vi "Keithley 6514 Resistance Config.vi"(0 "Resource In":refnum<visa-resource-name>, 1 "Check For SCPI Errors? (T)":bool=TRUE, 5 "range (autorange:0)":u16(ring) items=["autorange", "set min range", "set max range", "set man range value"], 7 "NPLC value (1.00)":dbl=1.0 min=0.01 max=10.0 step=0.01 format="%.2f", 9 "man range value (ohms) (210e3)":sgl=210000.0 min=0 max=2.1e+11 step=1 format="%^.2e", 11 "error in (no error)":T1, 12 "Autorange Upper Limit (ohms) (210e9)":sgl=210000000000.0 min=0 max=2.1e+11 step=1 format="%^.2e", 13 "Autorange Lower Limit (ohms) (2.1e3)":sgl=2100.0 min=0 max=2.1e+11 step=1 format="%^.2e", 14 "Driven Guard":bool) -> (4 "Resource Out (dupl)":refnum<visa-resource-name>, 15 "error out":T1)   [LabVIEW 2014, in "KE6514Driver.lvlib"]
doc: "This VI is used to configure the settings for resistance measurements.\n\nNPLC:\n0.01 to 10\n\nDriven Guard:\nTRUE = on\nFALSE = Off\n\nRange:\n0 = Autoranging\n1 = Set minimum range\n2 = Set maximum range\n3 = Set range by value\n\nRange value:\n0 to 2.1e11\n\nAutorange Upper Limit:\n0 to 2.1e11 (2.1e11 default)\n\nAutorange Lower Limit:\n0 to 2.1e11 (2.1e3 default)"
uses:
  KE6514Driver.lvlib
panel:
  # "on\noff"
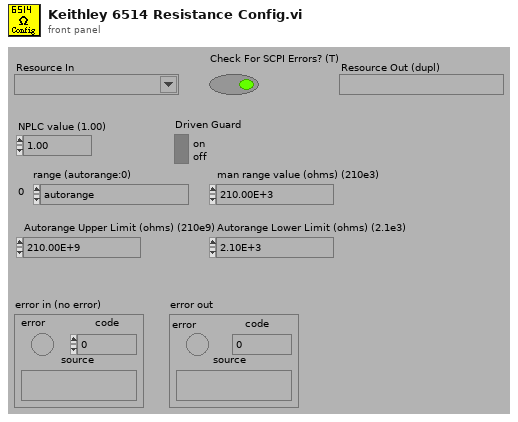
[diagram p1: front panel]
types:
  T1 = cluster{"error":bool, "code":i32, "source":string}
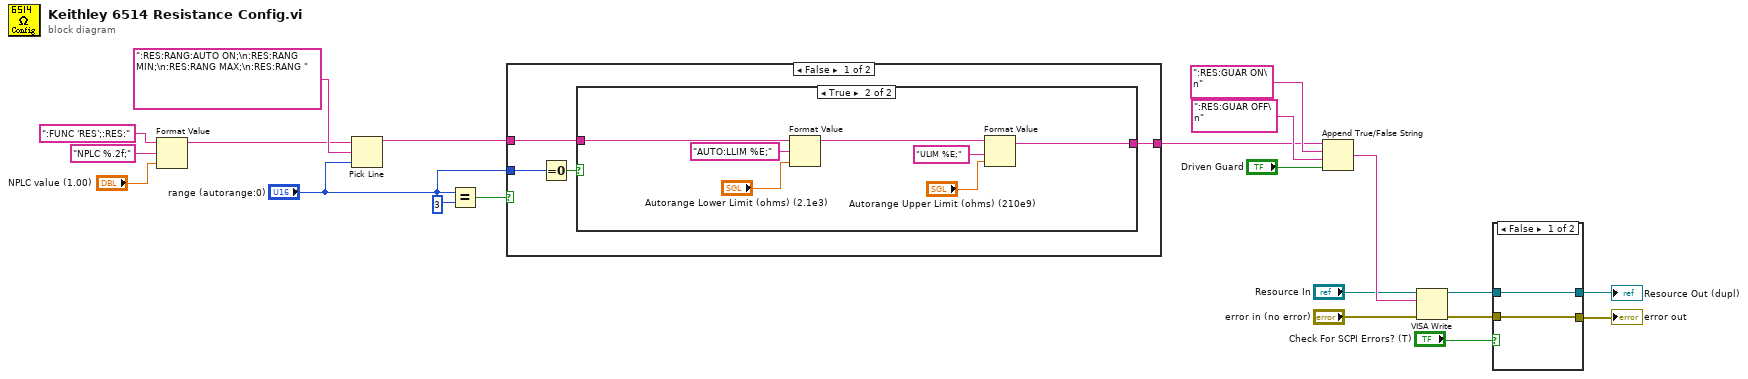
[diagram p0: block diagram]
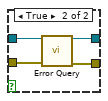
[diagram p2: hidden frame]
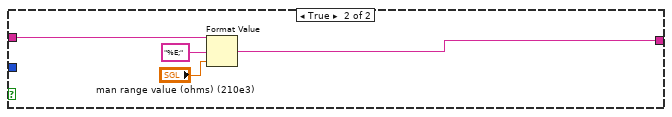
[diagram p4: hidden frame]
diagram:
  n1 = Format Value(string ("")=":FUNC 'RES';:RES:", format string="NPLC %.2f;", value (0)="NPLC value (1.00)") -> (output string=w11:string)
  n2 = Pick Line(string ("")=w11, multi-line string=":RES:RANG:AUTO ON;\n:RES:RANG MIN;\n:RES:RANG MAX;\n:RES:RANG ", line index="range (autorange:0)") -> (output string=w21:string)
  n3 = Equal?(x="range (autorange:0)", y=u16 3) -> (x = y?=w20:bool)
  n4 = case shown="False" w20 {
    tunnel: w21 -> [w24 w36]
    tunnel: [w25 w35] -> w10
    tunnel: "range (autorange:0)" -> [w22 _]
    frame False {
      n5 = Equal To 0?(x=w22) -> (x = 0?=w23:bool)
      n6 = case shown="True" w23 {
        tunnel: [w26 w32] -> w25
        tunnel: w24 -> [w26 w29]
        frame False {
        }
        frame True {
          n7 = Format Value(string ("")=w29, format string="AUTO:LLIM %E;", value (0)="Autorange Lower Limit (ohms) (2.1e3)") -> (output string=w33:string)
          n8 = Format Value(string ("")=w33, format string="ULIM %E;", value (0)="Autorange Upper Limit (ohms) (210e9)") -> (output string=w32:string)
        }
      }
    }
    frame True {
      n9 = Format Value(string ("")=w36, format string="%E;", value (0)="man range value (ohms) (210e3)") -> (output string=w35:string)
    }
  }
  n10 = Append True/False String(1:"Driven Guard", 2:":RES:GUAR OFF\n", 3:":RES:GUAR ON\n", 4:w10) -> (0:w8:string)
  n11 = VISA Write(VISA resource name="Resource In", write buffer=w8, error in (no error)="error in (no error)") -> (VISA resource name out=w4:refnum<visa-resource-name>, error out=w3:errorcluster)  [unwired: 1 out]
  n12 = case shown="False" "Check For SCPI Errors? (T)" {
    tunnel: w4 -> [w39 w43]
    tunnel: w3 -> [w38 w42]
    tunnel: [w38 w41] -> w2
    tunnel: [w39 w40] -> w1
    frame False {
    }
    frame True {
      n13 = call "Error Query.vi"("VISA Resource In"=w43, "error in (no error)"=w42) -> ("VISA Resource Out (dupl)"=w40:refnum<visa-resource-name>, "error out"=w41:errorcluster)  [unwired: 10 in, 2 out]
    }
  }
  "error out" <- w2
  "Resource Out (dupl)" <- w1
